vi "Read from LPC.vi"(0 "VISA resource name":refnum<visa-resource-name>="GPIB0::3::INSTR", 11 "error in (no error)":errorcluster) -> (3 "power":dbl[unit], 4 "VISA resource name out":refnum<visa-resource-name>, 6 "wavelength":dbl[unit], 8 "Transmission":dbl, 10 "control mode":T1(ring), 14 "front-panel controls":enum16{"enabled", "disabled"}(ring), 15 "error out":errorcluster)   [LabVIEW 2009, in "BEOC LPC.lvlib"]
doc: "Reads the most important settings from the LPC (laser power controller)."
uses:
  BEOC LPC.lvlib
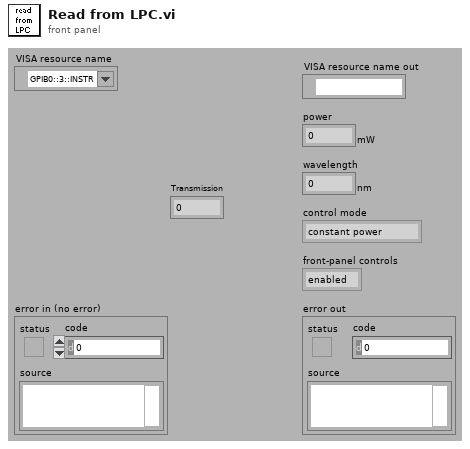
[diagram p1: front panel]
types:
  T1 = enum16{"constant power", "constant transmission"}
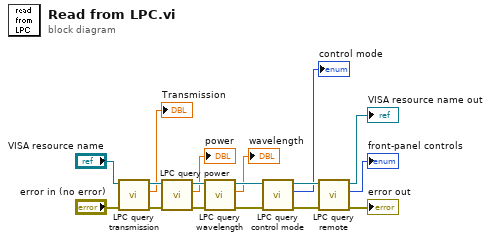
[diagram p0: block diagram]
diagram:
  n1 = call "LPC query transmission.vi"("error in (no error)"="error in (no error)", "VISA resource name"="VISA resource name") -> ("error out"=w4:errorcluster, "transmission (%)"=→"Transmission":dbl, "VISA resource name out"=w2:refnum<visa-resource-name>)  [unwired: 7 in]
  n2 = call "LPC query power.vi"("error in (no error)"=w4, "VISA resource name"=w2) -> ("error out"=w17:errorcluster, "power"=→"power":dbl[unit], "VISA resource name out"=w14:refnum<visa-resource-name>)  [unwired: 7 out]
  n3 = call "LPC query wavelength.vi"("error in (no error)"=w17, "VISA resource name"=w14) -> ("error out"=w16:errorcluster, "wavelength"=→"wavelength":dbl[unit], "VISA resource name out"=w13:refnum<visa-resource-name>)  [unwired: 7 out]
  n4 = call "LPC query control mode.vi"("error in (no error)"=w16, "VISA resource name"=w13) -> ("error out"=w15:errorcluster, "control mode"=→"control mode":T1, "VISA resource name out"=w12:refnum<visa-resource-name>)  [unwired: 7 out]
  n5 = call "LPC query remote.vi"("error in (no error)"=w15, "VISA resource name"=w12) -> ("error out"=→"error out":errorcluster, "front-panel controls"=→"front-panel controls":enum16{"enabled", "disabled"}, "VISA resource name out"=→"VISA resource name out":refnum<visa-resource-name>)  [unwired: 7 out]
